vi "多参数校准写入.vi"(8 "Error in":errorcluster caption="Error in (no error)", 9 "B":dbl caption="校准值B:", 10 "K":dbl caption="校准值K:", 11 "站号":u16(ring)=10 items=["氨氮"=3, "水温"=9, "pH值"=10, "溶解氧"=11, "电导率"=12, "浊度"=13, "叶绿素a"=14, "藻密度"=15, "蓝绿藻"=16, "氧化还原电位"=17, "溶解氧%"=18, "盐度"=19]) -> (0 "error out":errorcluster)   [LabVIEW 2016, in "斯坦道原位多参数.lvlib"]
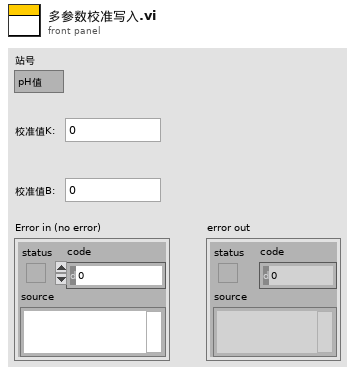
[diagram p1: front panel]
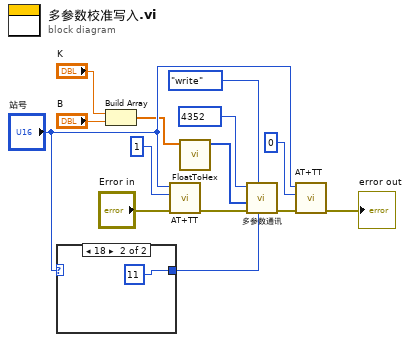
[diagram p0: block diagram]
diagram:
  n1 = case shown="18" "站号" {
    selector: "站号" -> [w15 _]
    tunnel: [w15 u16 11 ("站号")] -> w2
    frame 0, Default {
    }
    frame 18 {
    }
  }
  n2 = Build Array("K", "B") -> (w1:dbl[])
  n3 = call "AT+TT.vi"("错误输入（无错误）"="Error in", "Count"=1, "站号"="站号") -> ("错误输出"=w8:errorcluster)  [unwired: 7 in, 1 out]
  n4 = call "FloatToHex.vi"("浮点数"=w1) -> ("DCBA整形输出"=w12:u16[])  [unwired: 10 in]
  n5 = call "多参数通讯.vi"("Slave ID"=w2, "STEP"=enum16{"open", "read", "write", "close"}."write", "Error in"=w8, "values"=w12, "starting address"=u16 4352) -> ("error out"=w7:errorcluster)  [unwired: 4 in, 2 out]
  n6 = call "AT+TT.vi"("错误输入（无错误）"=w7, "Count"=0, "站号"="站号") -> ("错误输出"=→"error out":errorcluster)  [unwired: 7 in, 1 out]
